vi "Result.Numeric, Convert EV1 to EV2 Format.vi"(11 "Num EV1":T1[](array[typedef]) {"Status" items=["LOG", "PASS", "FAIL", "ERROR"]}) -> (3 "Num EV2":T4[](array[typedef]) {"Status" items=["LOG", "PASS", "FAIL", "ERROR"]})   [LabVIEW 2019]
uses:
  Result.Numeric.ctl
  Result.Limit Type.ctl
  Result.Measurement and Attribute Item Status.ctl
  Result.Numeric_EV1.ctl
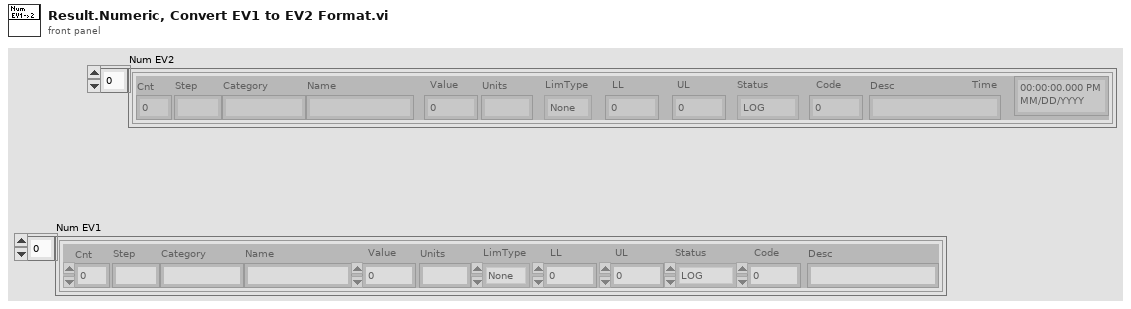
[diagram p1: front panel]
types:
  T1 = typedef "Result.Numeric_EV1.ctl" = cluster{"Cnt":i32, "Step":string, "Category":string, "Name":string, "Value":dbl, "Units":string, "LimType":T2, "LL":dbl, "UL":dbl, "Status":T3, "Code":i32, "Desc":string}
  T2 = typedef "Result.Limit Type.ctl" = enum16{"None", "EQ", "NE", "GT", "LT", "GE", "LE", "GTLT", "GELE", "GELT", "GTLE", "LTGT", "LEGE", "LEGT", "LTGE", "Contains", "NotContains"}
  T3 = typedef "Result.Measurement and Attribute Item Status.ctl" = i32
  T4 = typedef "Result.Numeric.ctl" = cluster{"Cnt":i32, "Step":string, "Category":string, "Name":string, "Value":dbl, "Units":string, "LimType":T2, "LL":dbl, "UL":dbl, "Status":T3, "Code":i32, "Desc":string, "Time":timestamp}
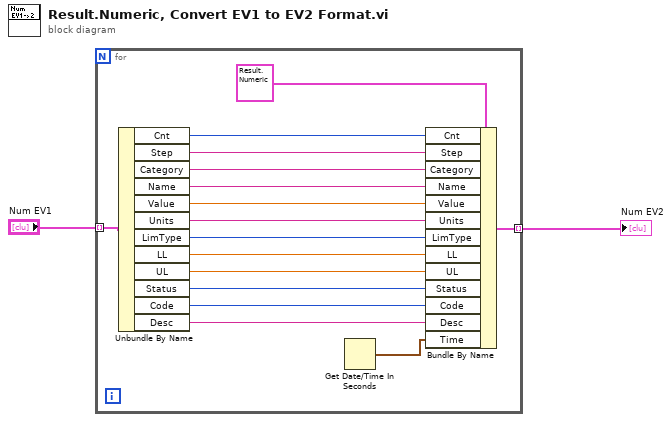
[diagram p0: block diagram]
diagram:
  n1 = for {
    tunnel: "Num EV1" -> [w18] mode=indexing
    tunnel: [w16] -> w1 mode=indexing
    n2 = Unbundle By Name(w18) -> ("Cnt"=w15:i32, "Step"=w14:string, "Category"=w13:string, "Name"=w12:string, "Value"=w11:dbl, "Units"=w10:string, "LimType"=w9:T2, "LL"=w8:dbl, "UL"=w7:dbl, "Status"=w6:T3, "Code"=w5:i32, "Desc"=w4:string)
    n3 = Get Date/Time In Seconds() -> (seconds since 1Jan1904=w3:timestamp)
    n4 = Bundle By Name(cluster=T4 {"Cnt"=0, "Step"="", "Category"="", "Name"="", "Value"=0.0, "Units"="", "LimType"=enum."None", "LL"=0.0, "UL"=0.0, "Status"=0, "Code"=0, "Desc"="", "Time"=timestamp(0 s since 1904-01-01)} ("Measurement"), "Cnt"=w15, "Step"=w14, "Category"=w13, "Name"=w12, "Value"=w11, "Units"=w10, "LimType"=w9, "LL"=w8, "UL"=w7, "Status"=w6, "Code"=w5, "Desc"=w4, "Time"=w3) -> (w16:T4)
  }
  "Num EV2" <- w1
